vi "Lab2_1.vi"() -> ()   [LabVIEW 2021]
panel:
  in  "InputX":sgl
  out "N!":i64
  in  "Stepen":i64
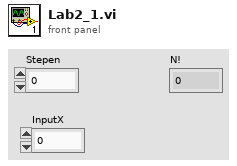
[diagram p1: front panel]
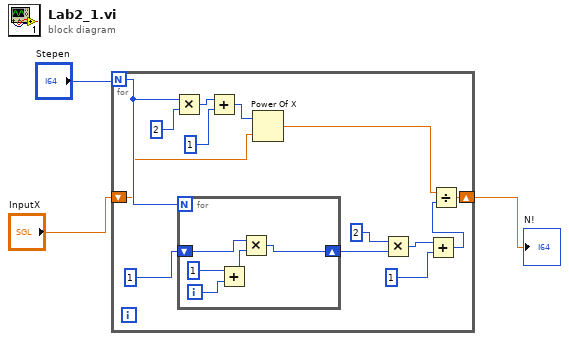
[diagram p0: block diagram]
diagram:
  n1 = for {
    N: "Stepen" -> [w10]
    shift-right: [w11] -> w3
    shift-left: "InputX" -> [w5]
    n2 = Multiply(x=w10, y=2) -> (x*y=w7:i32)
    n3 = for {
      N: w10 -> [_]
      shift-right: [w20] -> w16
      shift-left: 1 -> [w18]
      i -> [w22]
      n4 = Add(x=1, y=w22) -> (x+y=w21:i32)
      n5 = Multiply(x=w18, y=w21) -> (x*y=w20:i32)
    }
    n6 = Add(x=w7, y=1) -> (x+y=w6:i32)
    n7 = Power Of X(1:w5, 2:w6) -> (0:w4:sgl)
    n8 = Multiply(x=2, y=w16) -> (x*y=w14:i32)
    n9 = Add(x=w14, y=1) -> (x+y=w12:i32)
    n10 = Divide(x=w4, y=w12) -> (x/y=w11:sgl)
  }
  "N!" <- w3
